vi "createDirectory.vi"(8 "error in (no error)":errorcluster, 10 "targetBasePath":path, 11 "Module in":refnum<class "Module.lvclass">) -> (0 "error out":errorcluster, 2 "directoryPath":path, 3 "Module out":refnum<class "Module.lvclass">)   [LabVIEW 2013, in "Module.lvclass"]
uses:
  Module.lvclass
  Module.lvclass/Module.ctl
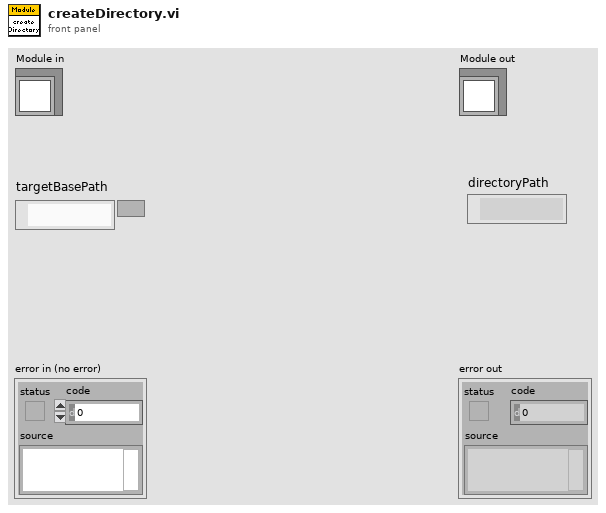
[diagram p1: front panel]
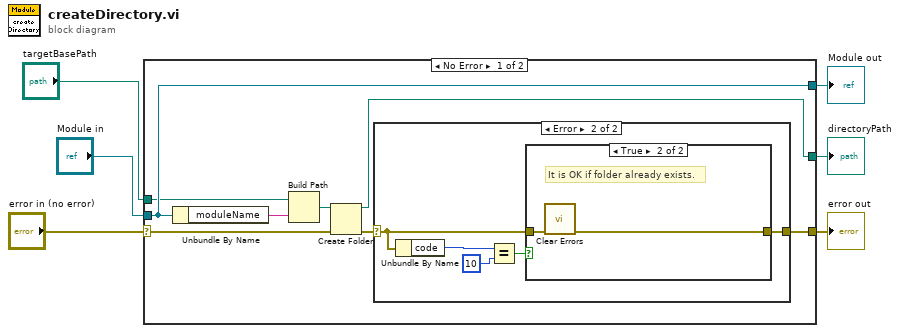
[diagram p0: block diagram]
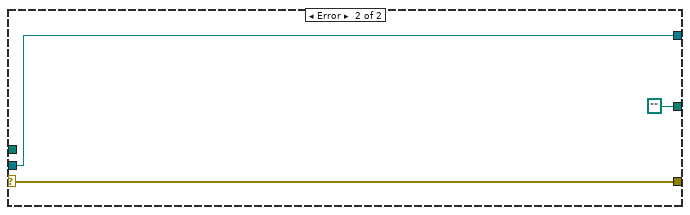
[diagram p4: hidden frame]
diagram:
  n1 = case shown="No Error" "error in (no error)" {
    selector: "error in (no error)" -> [w8 w26]
    tunnel: [w9 w26] -> w5
    tunnel: [w12 w25] -> w3
    tunnel: "Module in" -> [w12 w25]
    tunnel: "targetBasePath" -> [w10 _]
    tunnel: [w7 path ""] -> w1
    frame No Error {
      n2 = Unbundle By Name(w12) -> ("moduleName"=w11:string)
      n3 = Build Path(base path=w10, name or relative path=w11) -> (appended path=w14:path)
      n4 = Create Folder(path (use dialog)=w14, error in=w8) -> (created path=w7:path, error out=w13:errorcluster)  [unwired: 1 in, 1 out]
      n5 = case shown="Error" w13 {
        selector: w13 -> [w15 w18]
        tunnel: [w15 w17] -> w9
        frame No Error {
        }
        frame Error {
          n6 = Unbundle By Name(w18) -> ("code"=w20:i32)
          n7 = Equal?(x=w20, y=10) -> (x = y?=w16:bool)
          n8 = case shown="True" w16 {
            tunnel: w18 -> [w21 w23]
            tunnel: [w21 w22] -> w17
            frame False {
            }
            frame True {
              # "It is OK if folder already exists."
              n9 = call <vilib>:"Clear Errors.vi"("error in (no error)"=w23) -> ("error out"=w22:errorcluster)  [unwired: 6 in]
            }
          }
        }
      }
    }
    frame Error {
    }
  }
  "error out" <- w5
  "Module out" <- w3
  "directoryPath" <- w1
